vi "Set Data_To_Encrypt.vi"(8 "error in (no error)":errorcluster caption="entrée d'erreur (pas d'erreur)", 10 "Data_To_Encrypt":string, 11 "Cryptographic Hash (Default) en entrée":refnum<class "Cryptographic Hash (Default).lvclass">) -> (0 "error out":errorcluster caption="sortie d'erreur", 3 "Cryptographic Hash (Default) en sortie":refnum<class "Cryptographic Hash (Default).lvclass">)   [LabVIEW 2020, in "Library Cryptographic Hash.lvlib" / "Cryptographic Hash (Default).lvclass"]
uses:
  Cryptographic Hash (Default).lvclass
  Cryptographic Hash (Default).lvclass/Cryptographic Hash (Default).ctl
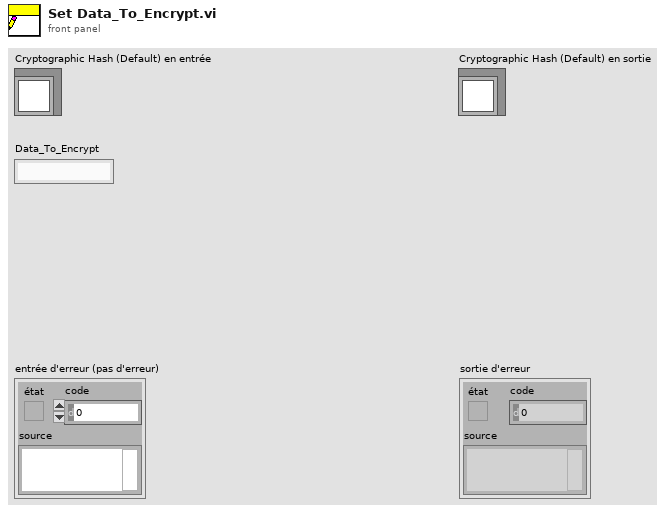
[diagram p1: front panel]
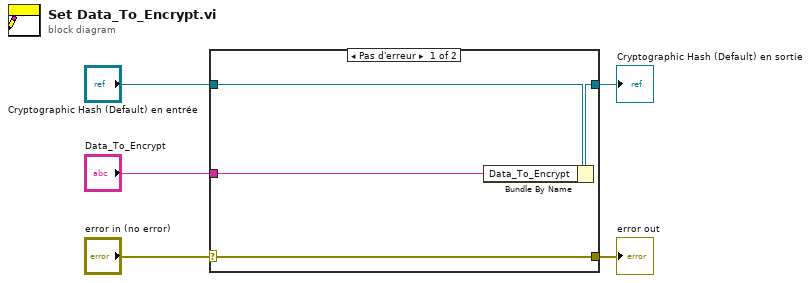
[diagram p0: block diagram]
diagram:
  n1 = case shown="Pas d'erreur" "error in (no error)" {
    selector: "error in (no error)" -> [w9 w10]
    tunnel: [w9 w10] -> w4
    tunnel: [w7 w11] -> w2
    tunnel: "Cryptographic Hash (Default) en entrée" -> [w8 w11]
    tunnel: "Data_To_Encrypt" -> [w6 _]
    frame No Error {
      n2 = Bundle By Name(cluster=w8, "Data_To_Encrypt"=w6) -> (w7:refnum<class "Cryptographic Hash (Default).lvclass">)
    }
    frame Error {
    }
  }
  "error out" <- w4
  "Cryptographic Hash (Default) en sortie" <- w2
